vi "Write Voltage.vi"(8 "error in (no error)":errorcluster, 10 "Voltage":dbl, 11 "Update Fan Voltage MSG in":refnum<class "Update Fan Voltage MSG.lvclass">) -> (0 "error out":errorcluster, 3 "Update Fan Voltage MSG out":refnum<class "Update Fan Voltage MSG.lvclass">)   [LabVIEW 2017, in "Controller.lvlib" / "Update Fan Voltage MSG.lvclass"]
uses:
  Update Fan Voltage MSG.lvclass
  Update Fan Voltage MSG.lvclass/Update Fan Voltage MSG.ctl
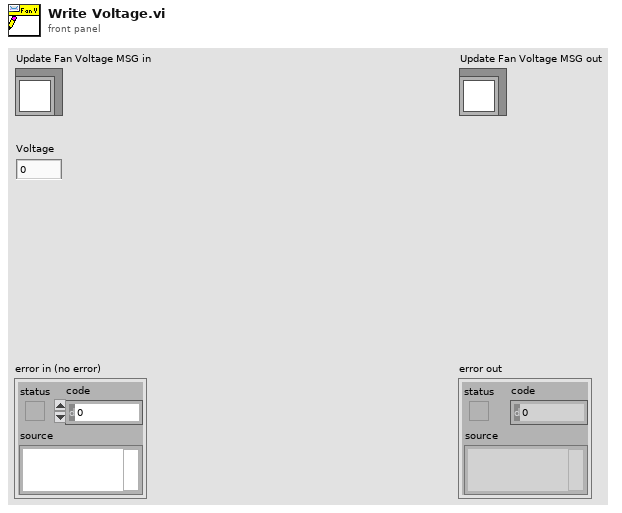
[diagram p1: front panel]
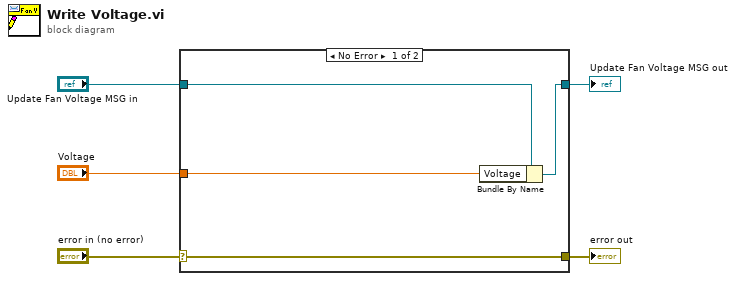
[diagram p0: block diagram]
diagram:
  n1 = case shown="No Error" "error in (no error)" {
    selector: "error in (no error)" -> [w9 w10]
    tunnel: [w9 w10] -> w4
    tunnel: [w7 w11] -> w2
    tunnel: "Update Fan Voltage MSG in" -> [w8 w11]
    tunnel: "Voltage" -> [w6 _]
    frame No Error {
      n2 = Bundle By Name(cluster=w8, "Voltage"=w6) -> (w7:refnum<class "Update Fan Voltage MSG.lvclass">)
    }
    frame Error {
    }
  }
  "error out" <- w4
  "Update Fan Voltage MSG out" <- w2
